vi "Rd Wr Lakeshore 336 settings json.vi"(8 "error in (no error)":errorcluster, 9 "Settings File":string="CC System Settings.json", 10 "Write? (F:Read)":bool, 11 "Lakeshore 336 Settings":T1={"Lake Shore 336 Address"="TCPIP0::192.168.121.12::7777::SOCKET", "Output Ch"=[{"Input (0:None)"=1, "Power Up Enable (F: Off)"=FALSE, "Mode (0:Off)"=0, "Max Current (0:User Specified)"=0, "Heater Out Display (1:Current)"=1, "Max User Current (2.000)"=2.0, "Heater Resistance (1:25 Ohms)"=2, "PID"={"P"=0.0, "I"=0.0, "D"=0.0}, "Name"="Output 1"}, {"Input (0:None)"=2, "Power Up Enable (F: Off)"=FALSE, "Mode (0:Off)"=0, "Max Current (0:User Specified)"=0, "Heater Out Display (1:Current)"=1, "Max User Current (2.000)"=2.0, "Heater Resistance (1:25 Ohms)"=2, "PID"={"P"=0.0, "I"=0.0, "D"=0.0}, "Name"="Output 2"}], "Input Ch"=[{"Name"="Input A"}, {"Name"="Input B"}, {"Name"="Input C"}, {"Name"="Input D"}], "Prefix"="LS336", "Setpoints"=[280.0, 280.0], "Control Enable"=[FALSE, FALSE]} {"Output Ch"."Heater Resistance (1:25 Ohms)" items=["25 Ohms"=1, "50 Ohms"=2]; "Output Ch"."Max User Current (2.000)" format="%.3f"; "Output Ch"."Heater Out Display (1:Current)" items=["Current"=1, "Power"=2]; "Output Ch"."Max Current (0:User Specified)" items=["User Specified", "0.707 A", "1.0 A", "1.141 A", "2.0 A"]; "Output Ch"."Mode (0:Off)" items=["Off", "Closed Loop PID", "Zone", "Open Loop"]; "Output Ch"."Input (0:None)" items=["None", "A", "B", "C", "D"]}) -> (0 "error out":errorcluster, 3 "Lakeshore 336 Settings":T1={"Lake Shore 336 Address"="TCPIP0::192.168.121.12::7777::SOCKET", "Output Ch"=[], "Input Ch"=[], "Prefix"="", "Setpoints"=[], "Control Enable"=[]} {"Output Ch"."Heater Resistance (1:25 Ohms)" items=["25 Ohms"=1, "50 Ohms"=2]; "Output Ch"."Max User Current (2.000)" format="%.3f"; "Output Ch"."Heater Out Display (1:Current)" items=["Current"=1, "Power"=2]; "Output Ch"."Max Current (0:User Specified)" items=["User Specified", "0.707 A", "1.0 A", "1.141 A", "2.0 A"]; "Output Ch"."Mode (0:Off)" items=["Off", "Closed Loop PID", "Zone", "Open Loop"]; "Output Ch"."Input (0:None)" items=["None", "A", "B", "C", "D"]})   [LabVIEW 2024, in "Lakeshore 336.lvclass"]
uses:
  Lakeshore 336.lvclass
  Lakeshore 336 Settings cluster.ctl
  Lakeshore 336 Channel Settings cluster.ctl
  Lakeshore 336 PID cluster.ctl
  Lakeshore 336 Input Ch config cluster.ctl
  2e80df6d-94aa-46b9-8b94-ceea8c057880.vi
  659fb017-0e9f-42f9-b06e-930303f00cbc.vi
  <vilib>/JDP Science/JSONtext/Find Item.vi
  <vilib>/JDP Science/JSONtext/Next JSON Value.vi
  <vilib>/JDP Science/JSONtext/String Subset.vi
  <vilib>/JDP Science/JSONtext/Parsing/Advance past next JSON Value (inlined COPY).vi
  <vilib>/JDP Science/JSONtext/Parsing/Advance past whitespace.vi
  <vilib>/JDP Science/JSONtext/Parsing/Advance past String.vi
  <vilib>/JDP Science/JSONtext/Parsing/Advance past Number.vi
  <vilib>/JDP Science/JSONtext/Parsing/Advance past Line Ending.vi
  <vilib>/JDP Science/JSONtext/Parsing/Parse Full Path or Item Name.vi
  <vilib>/JDP Science/JSONtext/Parsing/Advance past Array.vi
  <vilib>/JDP Science/JSONtext/Parsing/Advance past Object.vi
  <vilib>/JDP Science/JSONtext/support/Error Cluster From Code.vi
  <vilib>/JDP Science/JSONtext/Offset/Find Item Locations by Path.vi
  <vilib>/JDP Science/JSONtext/JSON text to Variant.vi
  <vilib>/JDP Science/JSONtext/Variant to JSON Text.vi
  <vilib>/JDP Science/JSONtext/Set Item.vi
  <vilib>/JDP Science/JSONtext/LVClass Serializer/JSONtext LVClass Serializer.lvclass
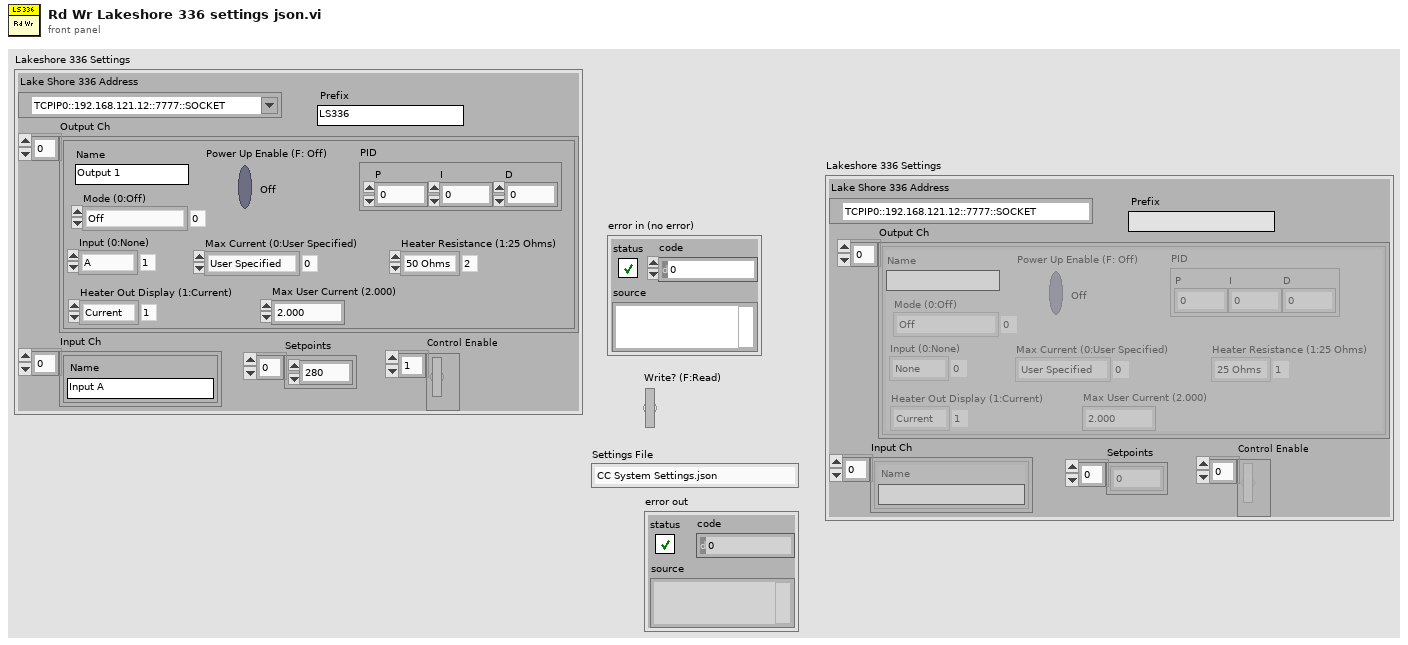
[diagram p1: front panel]
types:
  T1 = typedef "Lakeshore 336.lvclass/Lakeshore 336 Settings cluster.ctl" = cluster{"Lake Shore 336 Address":refnum<visa-resource-name>, "Output Ch":T2[], "Input Ch":T4[], "Prefix":string, "Setpoints":dbl[], "Control Enable":bool[]}
  T2 = typedef "Lakeshore 336.lvclass/Lakeshore 336 Channel Settings cluster.ctl" = cluster{"Input (0:None)":u16, "Power Up Enable (F: Off)":bool, "Mode (0:Off)":u16, "Max Current (0:User Specified)":u16, "Heater Out Display (1:Current)":u16, "Max User Current (2.000)":dbl, "Heater Resistance (1:25 Ohms)":u16, "PID":T3, "Name":string}
  T3 = typedef "Lakeshore 336.lvclass/Lakeshore 336 PID cluster.ctl" = cluster{"P":dbl, "I":dbl, "D":dbl}
  T4 = typedef "Lakeshore 336.lvclass/Lakeshore 336 Input Ch config cluster.ctl" = cluster{"Name":string}
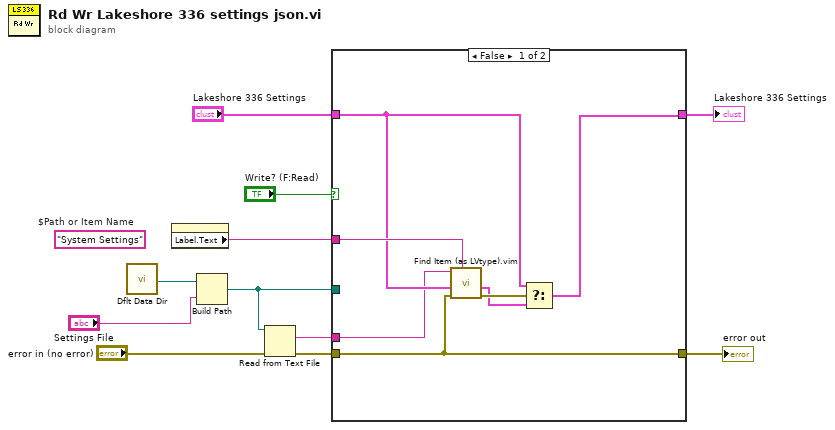
[diagram p0: block diagram]
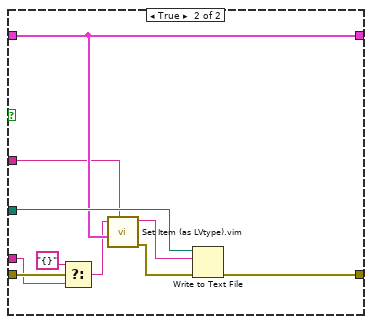
[diagram p2: hidden frame]
diagram:
  (unwired) "System Settings"  # $Path or Item Name
  n1 = call <vilib>:"Dflt Data Dir.vi"() -> ("App:Default Data Directory"=w8:path)
  n2 = property on="Lakeshore 336 Settings" class="Clust (strict)"() -> ("Label.Text"=w1:string)  [unwired: 2 in, 2 out]
  n3 = Build Path(base path=w8, name or relative path="Settings File") -> (appended path=w2:path)
  n4 = Read from Text File(file (use dialog)=w2, error in="error in (no error)") -> (text=w3:string, error out=w4:errorcluster)  [unwired: 2 in, 2 out]
  n5 = case shown="False" "Write? (F:Read)" {
    tunnel: w4 -> [w12 w23]
    tunnel: "Lakeshore 336 Settings" -> [w16 w26]
    tunnel: w2 -> [_ w28]
    tunnel: [w12 w27] -> w7
    tunnel: [w18 w26] -> w6
    tunnel: w1 -> [w17 w25]
    tunnel: w3 -> [w13 w21]
    frame False {
      n6 = call "Find Item (as LVtype).vim"("$Path or Item Name"=w17, "error in (no error)"=w12, "Data Type and Default Value"=w16, "JSON"=w13) -> ("error out"=w15:errorcluster, "Data"=w14:T1)  [unwired: 4 in, 2 out]
      n7 = Select(t=w16, s=w15, f=w14) -> (s? t:f=w18:T1)
    }
    frame True {
      n8 = Select(t="{}" ("JSON"), s=w23, f=w21) -> (s? t:f=w20:string)
      n9 = call "Set Item (as LVtype).vim"("$Path or Item Name"=w25, "Anything"=w26, "JSON"=w20) -> ("error out"=w19:errorcluster, "<JSON>"=w24:string)  [unwired: 5 in, 1 out]
      n10 = Write to Text File(file (use dialog)=w28, text=w24, error in=w19) -> (error out=w27:errorcluster)  [unwired: 1 in, 2 out]
    }
  }
  "error out" <- w7
  "Lakeshore 336 Settings" <- w6
